vi "AlliGator Select Phasor Calibration v3.vi"(0 "Calibration Phasor":T6={"m"=1.0, "phi"=0.0, "Phasor Frequency"=0.0, "Reference Lifetime"=0.0}, 1 "ROI Center (Default: undefined)":cluster{"X":i32, "Y":i32}={"X"=2147483647, "Y"=2147483647}, 2 "Basic Calibration Options":T1, 5 "Calibration Phasor Series":T7, 7 "Phasor Calibration Map":T4={"Phasor Frequency"=80000000.0, "Calibration Lifetime"=1e-09, "ROI Centers"=[], "ROI Descriptors"=[], "Map Resolution X"=0, "Map Resolution Y"=0, "z Array"=[]} {"ROI Descriptors"."Contours"."Type" items=["No Selection", "Point", "Line", "Rectangle", "Oval", "Polygon", "Freehand Region", "Annulus", "Unused2", "Unused3", "Broken Line", "Freehand Line", "Rotated Rectangle"]}, 9 "Calibration Map MD5 Digest":string, 11 "Error In":errorcluster, 12 "Current Data Set (-1: single)":i32=-1, 13 "Full-Frame Single-Pixel Calibration?":bool) -> (4 "Calibration Phasor":T6, 10 "Phasor Calibration Map Characteristics":T3={"Phasor Frequency"=80000000.0, "Calibration Lifetime"=1e-09, "Map Resolution X"=0, "Map Resolution Y"=0, "Empty Map"=FALSE}, 15 "Error Out":errorcluster)   [LabVIEW 2021, in "AlliGator Phasor Calibration.lvlib"]
doc: "Picks the appropriate Phasor Calibration, depending on the <B>ROI Center</B> and <B>Current Data Set</B> and phasor calibration options (single calibration, series or map)."
uses:
  AlliGator Phasor Calibration.lvlib
  Phasor/Phasor Reference Series.ctl
  Phasor/Calibration Phasor (m, phi).ctl
  Phasor/Phasor Calibration Map v2.ctl
  Phasor/Phasor Calibration Map Characteristics.ctl
  Phasor/Phasor.lvlib
  Phasor/Phasor Calibration Type.ctl
  AlliGator Basic Calibration Options .ctl
panel:
  # "see the AlliGator License on the block diagram (Ctrl+E or Window:Show Block Diagram)"
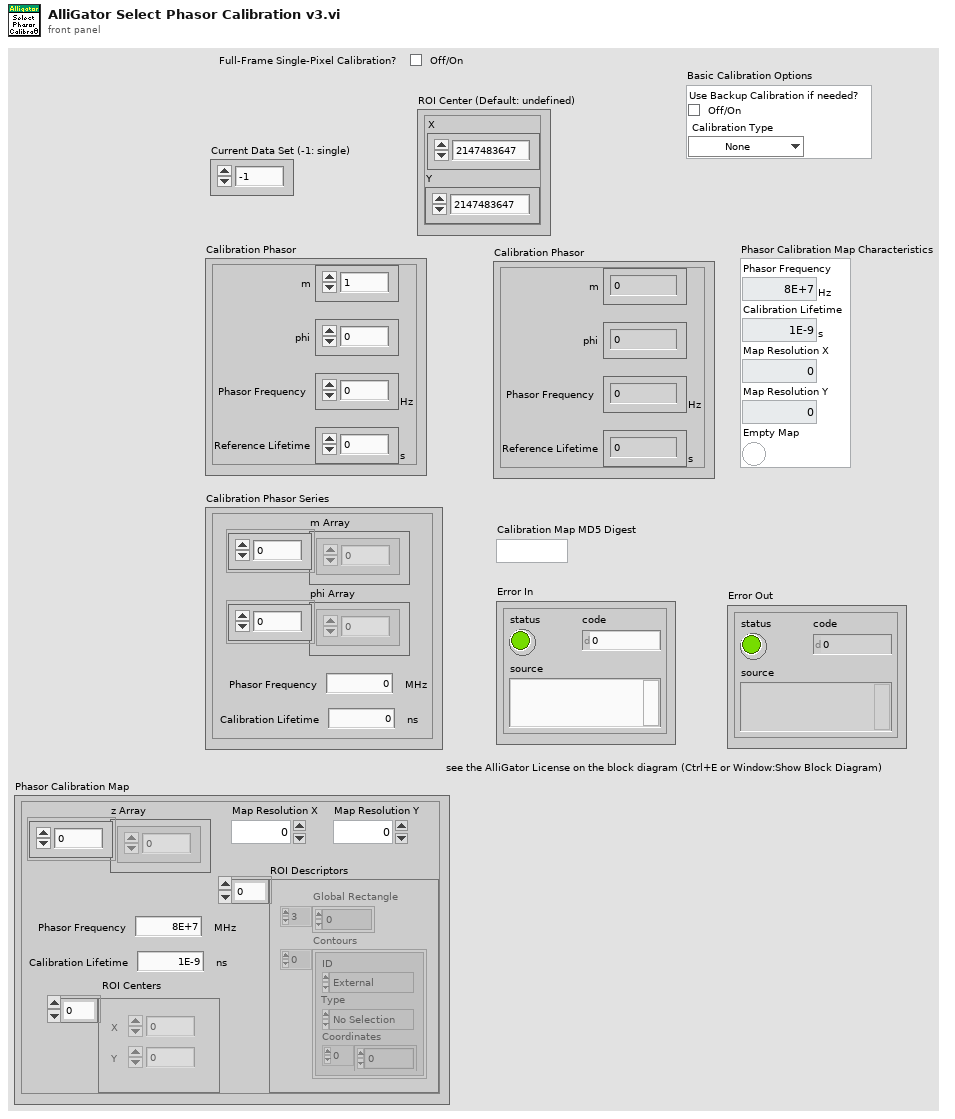
[diagram p1: front panel]
types:
  T1 = typedef "AlliGator Phasor Calibration.lvlib/AlliGator Basic Calibration Options .ctl" = cluster{"Use Backup Calibration if needed?":bool, "Calibration Type":T2}
  T2 = typedef "Phasor.lvlib/Phasor Calibration Type.ctl" = enum16{"None", "Single Phasor", "Phasor Series", "Phasor Map"}
  T3 = typedef "Phasor.lvlib/Phasor Calibration Map Characteristics.ctl" = cluster{"Phasor Frequency":dbl[unit], "Calibration Lifetime":dbl[unit], "Map Resolution X":i32, "Map Resolution Y":i32, "Empty Map":bool}
  T4 = typedef "Phasor.lvlib/Phasor Calibration Map v2.ctl" = cluster{"Phasor Frequency":dbl[unit], "Calibration Lifetime":dbl[unit], "ROI Centers":cluster{"X":i32, "Y":i32}[], "ROI Descriptors":T5[], "Map Resolution X":i32, "Map Resolution Y":i32, "z Array":cdb[]}
  T5 = typedef "ROI Descriptor" = cluster{"Global Rectangle":i32[], "Contours":cluster{"ID":enum32{"External", "Internal"}, "Type":u32, "Coordinates":i32[]}[]}
  T6 = typedef "Phasor.lvlib/Calibration Phasor (m, phi).ctl" = cluster{"m":dbl, "phi":dbl, "Phasor Frequency":dbl[unit], "Reference Lifetime":dbl[unit]}
  T7 = typedef "Phasor.lvlib/Phasor Reference Series.ctl" = cluster{"m Array":dbl[], "phi Array":dbl[], "Phasor Frequency":dbl[unit], "Calibration Lifetime":dbl[unit]}
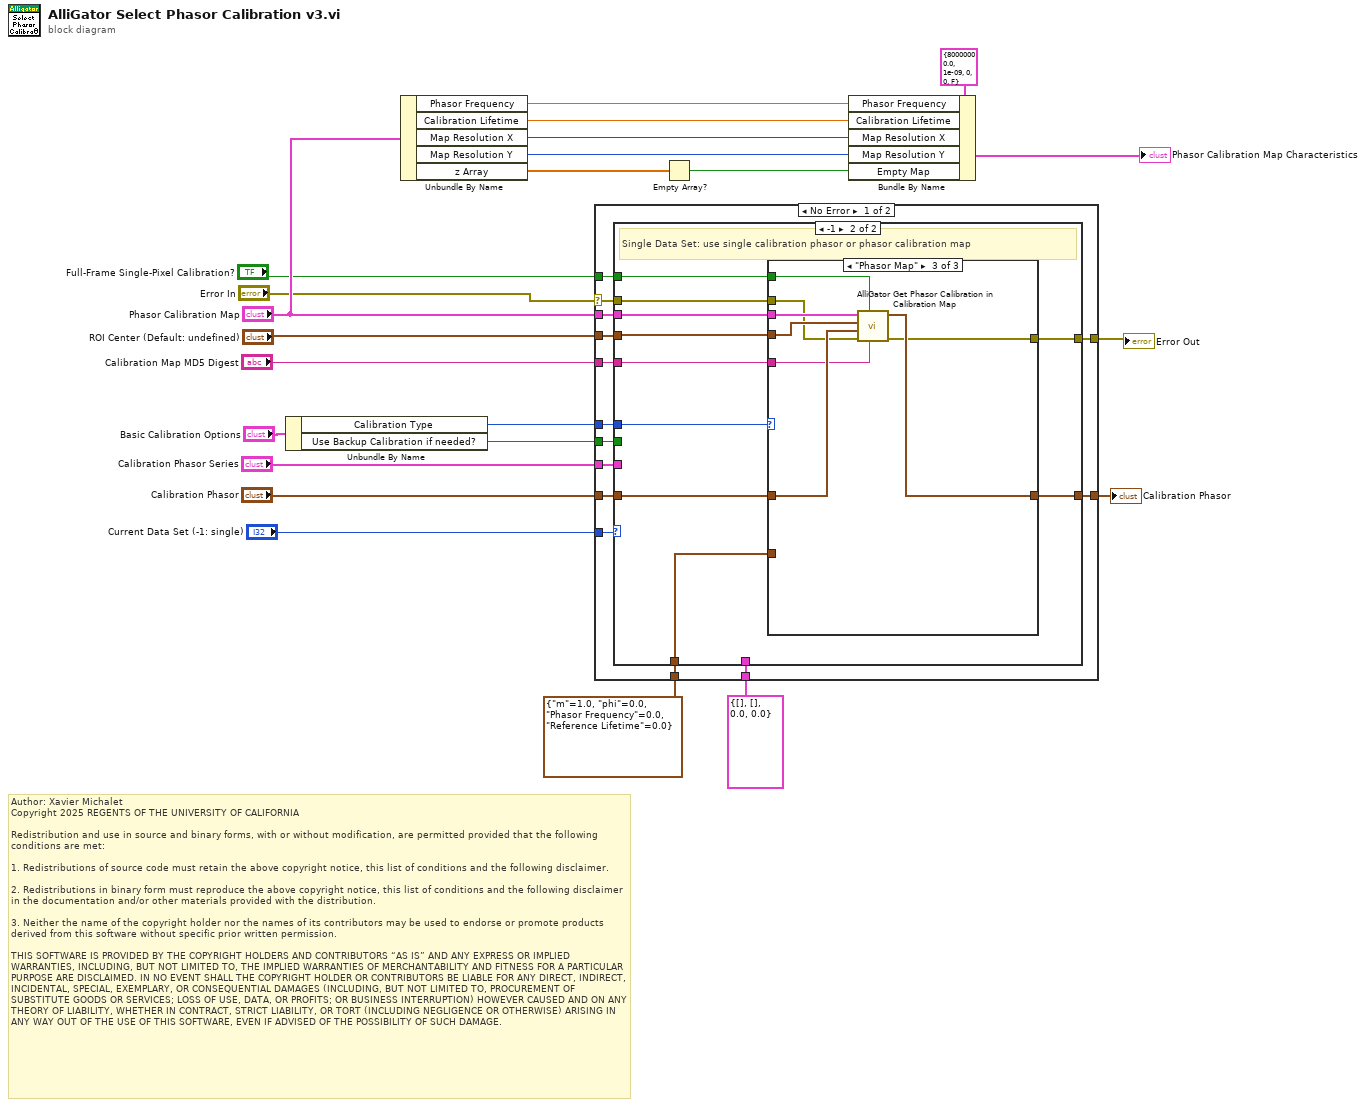
[diagram p0: block diagram]
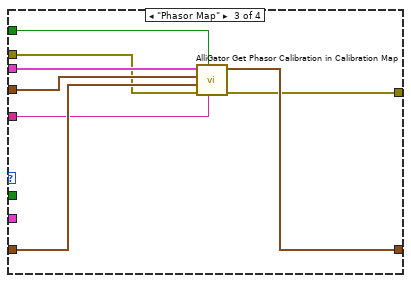
[diagram p4: hidden frame]
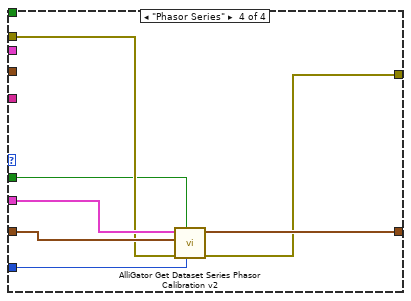
[diagram p5: hidden frame]
diagram:
  # "Author: Xavier Michalet\nCopyright 2025 REGENTS OF THE UNIVERSITY OF CALIFORNIA\n\nRedistribution and use in source and binary forms, with or without modification, are permitted provided that the following conditions are met:\n\n1. Redistributions of source code must retain the above copyright notice, this list of conditions and the following disclaimer.\n\n2. Redistributions in binary form must reproduce the above copyright notice, this list of conditions and the following disclaimer in the documentation and/or other materials provided with the distribution.\n\n3. Neither the name of the copyright holder nor the names of its contributors may be used to endorse or promote products derived from this software without specific prior written permission.\n\nTHIS SOFTWARE IS PROVIDED BY THE COPYRIGHT HOLDERS AND CONTRIBUTORS “AS IS” AND ANY EXPRESS OR IMPLIED WARRANTIES, INCLUDING, BUT NOT LIMITED TO, THE IMPLIED WARRANTIES OF MERCHANTABILITY AND FITNESS FOR A PARTICULAR PURPOSE ARE DISCLAIMED. IN NO EVENT SHALL THE COPYRIGHT HOLDER OR CONTRIBUTORS BE LIABLE FOR ANY DIRECT, INDIRECT, INCIDENTAL, SPECIAL, EXEMPLARY, OR CONSEQUENTIAL DAMAGES (INCLUDING, BUT NOT LIMITED TO, PROCUREMENT OF SUBSTITUTE GOODS OR SERVICES; LOSS OF USE, DATA, OR PROFITS; OR BUSINESS INTERRUPTION) HOWEVER CAUSED AND ON ANY THEORY OF LIABILITY, WHETHER IN CONTRACT, STRICT LIABILITY, OR TORT (INCLUDING NEGLIGENCE OR OTHERWISE) ARISING IN ANY WAY OUT OF THE USE OF THIS SOFTWARE, EVEN IF ADVISED OF THE POSSIBILITY OF SUCH DAMAGE."
  n1 = Unbundle By Name("Basic Calibration Options") -> ("Calibration Type"=w3:T2, "Use Backup Calibration if needed?"=w4:bool)
  n2 = Unbundle By Name("Phasor Calibration Map") -> ("Phasor Frequency"=w11:dbl[unit], "Calibration Lifetime"=w8:dbl[unit], "Map Resolution X"=w7:i32, "Map Resolution Y"=w6:i32, "z Array"=w10:cdb[])
  n3 = case shown="No Error" "Error In" {
    selector: "Error In" -> [w27 w93]
    tunnel: "Calibration Phasor Series" -> [w37 _]
    tunnel: "Calibration Phasor" -> [w36 _]
    tunnel: "Current Data Set (-1: single)" -> [w35 _]
    tunnel: [w34 w94] -> w20
    tunnel: T6 {"m"=1.0, "phi"=0.0, "Phasor Frequency"=0.0, "Reference Lifetime"=0.0} ("f") -> [w33 w94]
    tunnel: T7 {"m Array"=[], "phi Array"=[], "Phasor Frequency"=0.0, "Calibration Lifetime"=0.0} ("f") -> [w32 _]
    tunnel: "Phasor Calibration Map" -> [w31 _]
    tunnel: "ROI Center (Default: undefined)" -> [w30 _]
    tunnel: [w29 w93] -> w16
    tunnel: "Calibration Map MD5 Digest" -> [w28 _]
    tunnel: "Full-Frame Single-Pixel Calibration?" -> [w26 _]
    tunnel: w4 -> [w25 _]
    tunnel: w3 -> [w24 _]
    frame No Error {
      n4 = case shown="-1" w35 {
        selector: w35 -> [w51 _]
        tunnel: w36 -> [w50 w80]
        tunnel: [w46 w78] -> w34
        tunnel: w37 -> [w48 _]
        tunnel: w33 -> [w49 w79]
        tunnel: w32 -> [w47 _]
        tunnel: w31 -> [w45 w77]
        tunnel: w30 -> [w44 w76]
        tunnel: [w43 w75] -> w29
        tunnel: w28 -> [w42 w74]
        tunnel: w27 -> [w41 w73]
        tunnel: w26 -> [w40 w72]
        tunnel: w25 -> [w39 _]
        tunnel: w24 -> [w38 w71]
        frame 0, Default {
          # "Series: choice of calibration phasor source"
          n5 = case shown="\"None\", Default" w38 {
            tunnel: w51 -> [_ _ _ w70]
            tunnel: w50 -> [_ w55 w59 w66]
            tunnel: w49 -> [w53 _ _ _]
            tunnel: w48 -> [_ _ _ w69]
            tunnel: w47 -> [_ _ _ _]
            tunnel: [w53 w55 w63 w68] -> w46
            tunnel: w45 -> [_ _ w62 _]
            tunnel: w44 -> [_ _ w61 _]
            tunnel: [w52 w54 w60 w67] -> w43
            tunnel: w42 -> [_ _ w58 _]
            tunnel: w41 -> [w52 w54 w57 w65]
            tunnel: w40 -> [_ _ w56 _]
            tunnel: w39 -> [_ _ _ w64]
            frame "None", Default {
            }
            frame "Single Phasor" {
            }
            frame "Phasor Map" {
              n6 = call "AlliGator Get Phasor Calibration in Calibration Map.vi"("Calibration Map MD5 Digest"=w58, "Full-Frame Single-Pixel Calibration?"=w56, "Error In"=w57, "Phasor Calibration in"=w59, "ROI Center"=w61, "Phasor Calibration Map"=w62) -> ("Error Out"=w60:errorcluster, "Phasor Calibration out"=w63:T6)  [unwired: 4 in]
            }
            frame "Phasor Series" {
              n7 = call "AlliGator Get Dataset Series Phasor Calibration v2.vi"("Dataset Series Index"=w70, "Use Backup Calibration if needed?"=w64, "Error In"=w65, "Default Phasor Calibration"=w66, "Phasor Calibration Series"=w69) -> ("Error Out"=w67:errorcluster, "Phasor Calibration"=w68:T6)  [unwired: 5 in]
            }
          }
        }
        frame -1 {
          # "Single Data Set: use single calibration phasor or phasor calibration map"
          n8 = case shown="\"Phasor Map\"" w71 {
            tunnel: [w82 w84 w90] -> w78
            tunnel: w77 -> [_ _ w92]
            tunnel: w76 -> [_ _ w91]
            tunnel: [w81 w83 w89] -> w75
            tunnel: w80 -> [_ w84 w88]
            tunnel: w79 -> [w82 _ _]
            tunnel: w74 -> [_ _ w87]
            tunnel: w73 -> [w81 w83 w86]
            tunnel: w72 -> [_ _ w85]
            frame "None", Default {
            }
            frame "Single Phasor" {
            }
            frame "Phasor Map" {
              n9 = call "AlliGator Get Phasor Calibration in Calibration Map.vi"("Calibration Map MD5 Digest"=w87, "Full-Frame Single-Pixel Calibration?"=w85, "Error In"=w86, "Phasor Calibration in"=w88, "ROI Center"=w91, "Phasor Calibration Map"=w92) -> ("Error Out"=w89:errorcluster, "Phasor Calibration out"=w90:T6)  [unwired: 4 in]
            }
          }
        }
      }
    }
    frame Error {
    }
  }
  "Calibration Phasor" <- w20
  "Error Out" <- w16
  n10 = Empty Array?(array=w10) -> (empty?=w9:bool)
  n11 = Bundle By Name(cluster=T3 {"Phasor Frequency"=80000000.0, "Calibration Lifetime"=1e-09, "Map Resolution X"=0, "Map Resolution Y"=0, "Empty Map"=FALSE} ("Phasor Calibration Map Characteristics"), "Phasor Frequency"=w11, "Calibration Lifetime"=w8, "Map Resolution X"=w7, "Map Resolution Y"=w6, "Empty Map"=w9) -> (→"Phasor Calibration Map Characteristics":T3)
